vi "Periodic Tasks.vi"(8 "error in":errorcluster) -> ()   [LabVIEW 2019]
doc: "This VI runs in parallel to other tasks. It can contain as many user-defined periodic loops as you need. These can carry out PID or other sorts of timed response."
uses:
  <vilib>/Rock Robotics/WPI/Utilities/WPI_GetSetVariantRefNum.vi
  Robot Global Data.vi
  <vilib>/addons/control/pid/pid.llb/PID (DBL).vi
  <vilib>/Rock Robotics/Network Tables/NT Write Numeric Array.vi
  <vilib>/Rock Robotics/Network Tables/NT Write Number.vi
  <vilib>/Rock Robotics/Network Tables/NT Write Boolean.vi
  Secret_Control_Library_Protected/Secret_Control_Library_Protected.lvlib
  <vilib>/addons/control/pid/NI_PID_pid.lvlib
  <vilib>/Rock Robotics/WPI/ThirdParty/JAS_Junk/TrajLib/Trajectory_Library.lvlib
panel:
  in  "Speed PID":T1={"proportional gain (Kc)"=0.6, "integral time (Ti, min)"=0.015, "derivative time (Td, min)"=0.0} {"derivative time (Td, min)" format="%.3f"; "integral time (Ti, min)" format="%.3f"; "proportional gain (Kc)" format="%.3f"}
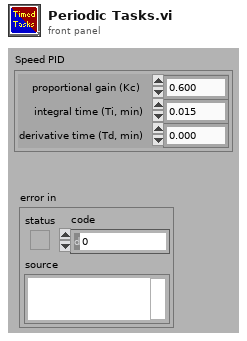
[diagram p1: front panel]
types:
  T1 = cluster{"proportional gain (Kc)":dbl, "integral time (Ti, min)":dbl, "derivative time (Td, min)":dbl}
  T2 = typedef "WPI_EncoderDevRef.ctl" = cluster{"DevStatus":errorcluster, "EncoderIndex":T3, "CounterIndex":T4, "DistancePerCount":dbl, "Decoding Type":T5}
  T3 = typedef "FPGA_EncoderIdx.ctl" = enum8{"Enc 0", "Enc 1", "Enc 2", "Enc 3", "Enc 4", "Enc 5", "Enc 6", "Enc 7", "Invalid"}
  T4 = typedef "FPGA_CounterCtrSystemIndex.ctl" = enum8{"Ctr 0", "Ctr 1", "Ctr 2", "Ctr 3", "Ctr 4", "Ctr 5", "Ctr 6", "Ctr 7", "Invalid"}
  T5 = typedef "WPI_EncoderType.ctl" = enum16{"1x", "2x", "4x"}
  T6 = typedef "WPI_GyroDevRef.ctl" = cluster{"DevStatus":errorcluster, "Analog Channel":T7, "Gain (VoltsPerDegree/Second)":dbl, "Gyro Type":enum16{"Analog", "XRS450"}, "Handle":i32, "SPI Bus":T8, "Device Found":bool, "Sample Rate":dbl, "Calibrate On Open":bool, "Offset":dbl}
  T7 = typedef "FPGA_AIChannel.ctl" = enum8{"AI 0", "AI 1", "AI 2", "AI 3", "AI MXP 0", "AI MXP 1", "AI MXP 2", "AI MXP 3", "Invalid"}
  T8 = typedef "spi_bus.ctl" = enum16{"SPI On-Board, CS0", "SPI On-Board, CS1", "SPI On-Board, CS2", "SPI On-Board, CS3", "SPI MXP", "Invalid"}
  T9 = typedef "WPI_RobotDriveDevRef.ctl" = cluster{"DevStatus":errorcluster, "Motors[]":T10[], "Square Inputs":bool, "Max Output":dbl}
  T10 = typedef "WPI_MotorControlDeviceRef.ctl" = cluster{"DeviceStatus":errorcluster, "Type":T11, "PWM":cluster{"PWM Channel":T12, "DeadBand":T13}, "CAN":cluster{"Device Number":u8, "SetOutput VI Ref":variant, "GetOutput VI Ref":variant, "Enable VI Ref":variant, "Disable VI Ref":variant, "Data":variant}, "Invert":bool, "DIO PWM":cluster{"PWM \"Enable\" Channel":T12, "DIOChannel":T14, "PWM Rate":dbl}}
  T11 = typedef "WPI_MotorControlType.ctl" = enum16{"PWM", "CAN", "DIO PWM"}
  T12 = typedef "FPGA_DIOPWMChannel.ctl" = enum8{"PWM 0", "PWM 1", "PWM 2", "PWM 3", "PWM 4", "PWM 5", "PWM 6", "PWM 7", "PWM 8", "PWM 9", "PWM MXP 0", "PWM MXP 1", "PWM MXP 2", "PWM MXP 3", "PWM MXP 4", "PWM MXP 5", "PWM MXP 6", "PWM MXP 7", "PWM MXP 8", "PWM MXP 9", "Invalid"}
  T13 = typedef "WPI_PWMDeadband.ctl" = cluster{"Name":string, "maxPositivePwm":i32, "minPositivePwm":i32, "centerPwm":i32, "maxNegativePwm":i32, "minNegativePwm":i32, "angularRange":u16}
  T14 = typedef "FPGA_DIOChannel.ctl" = enum8{"DIO 0", "DIO 1", "DIO 2", "DIO 3", "DIO 4", "DIO 5", "DIO 6", "DIO 7", "DIO 8", "DIO 9", "DIO MXP 0", "DIO MXP 1", "DIO MXP 2", "DIO MXP 3", "DIO MXP 4", "DIO MXP 5", "DIO MXP 6", "DIO MXP 7", "DIO MXP 8", "DIO MXP 9", "DIO MXP 10", "DIO MXP 11", "DIO MXP 12", "DIO MXP 13", "DIO MXP 14", "DIO MXP 15", "SPI Port CS1", "SPI Port CS2", "SPI Port CS3", "SPI Port MISO", "SPI Port MOSI", "Invalid"}
  T15 = typedef "Trajectory_Library.lvlib/SIMPLE_MOTOR_FF.ctl" = cluster{"Ks":dbl, "Kv":dbl, "Ka":dbl}
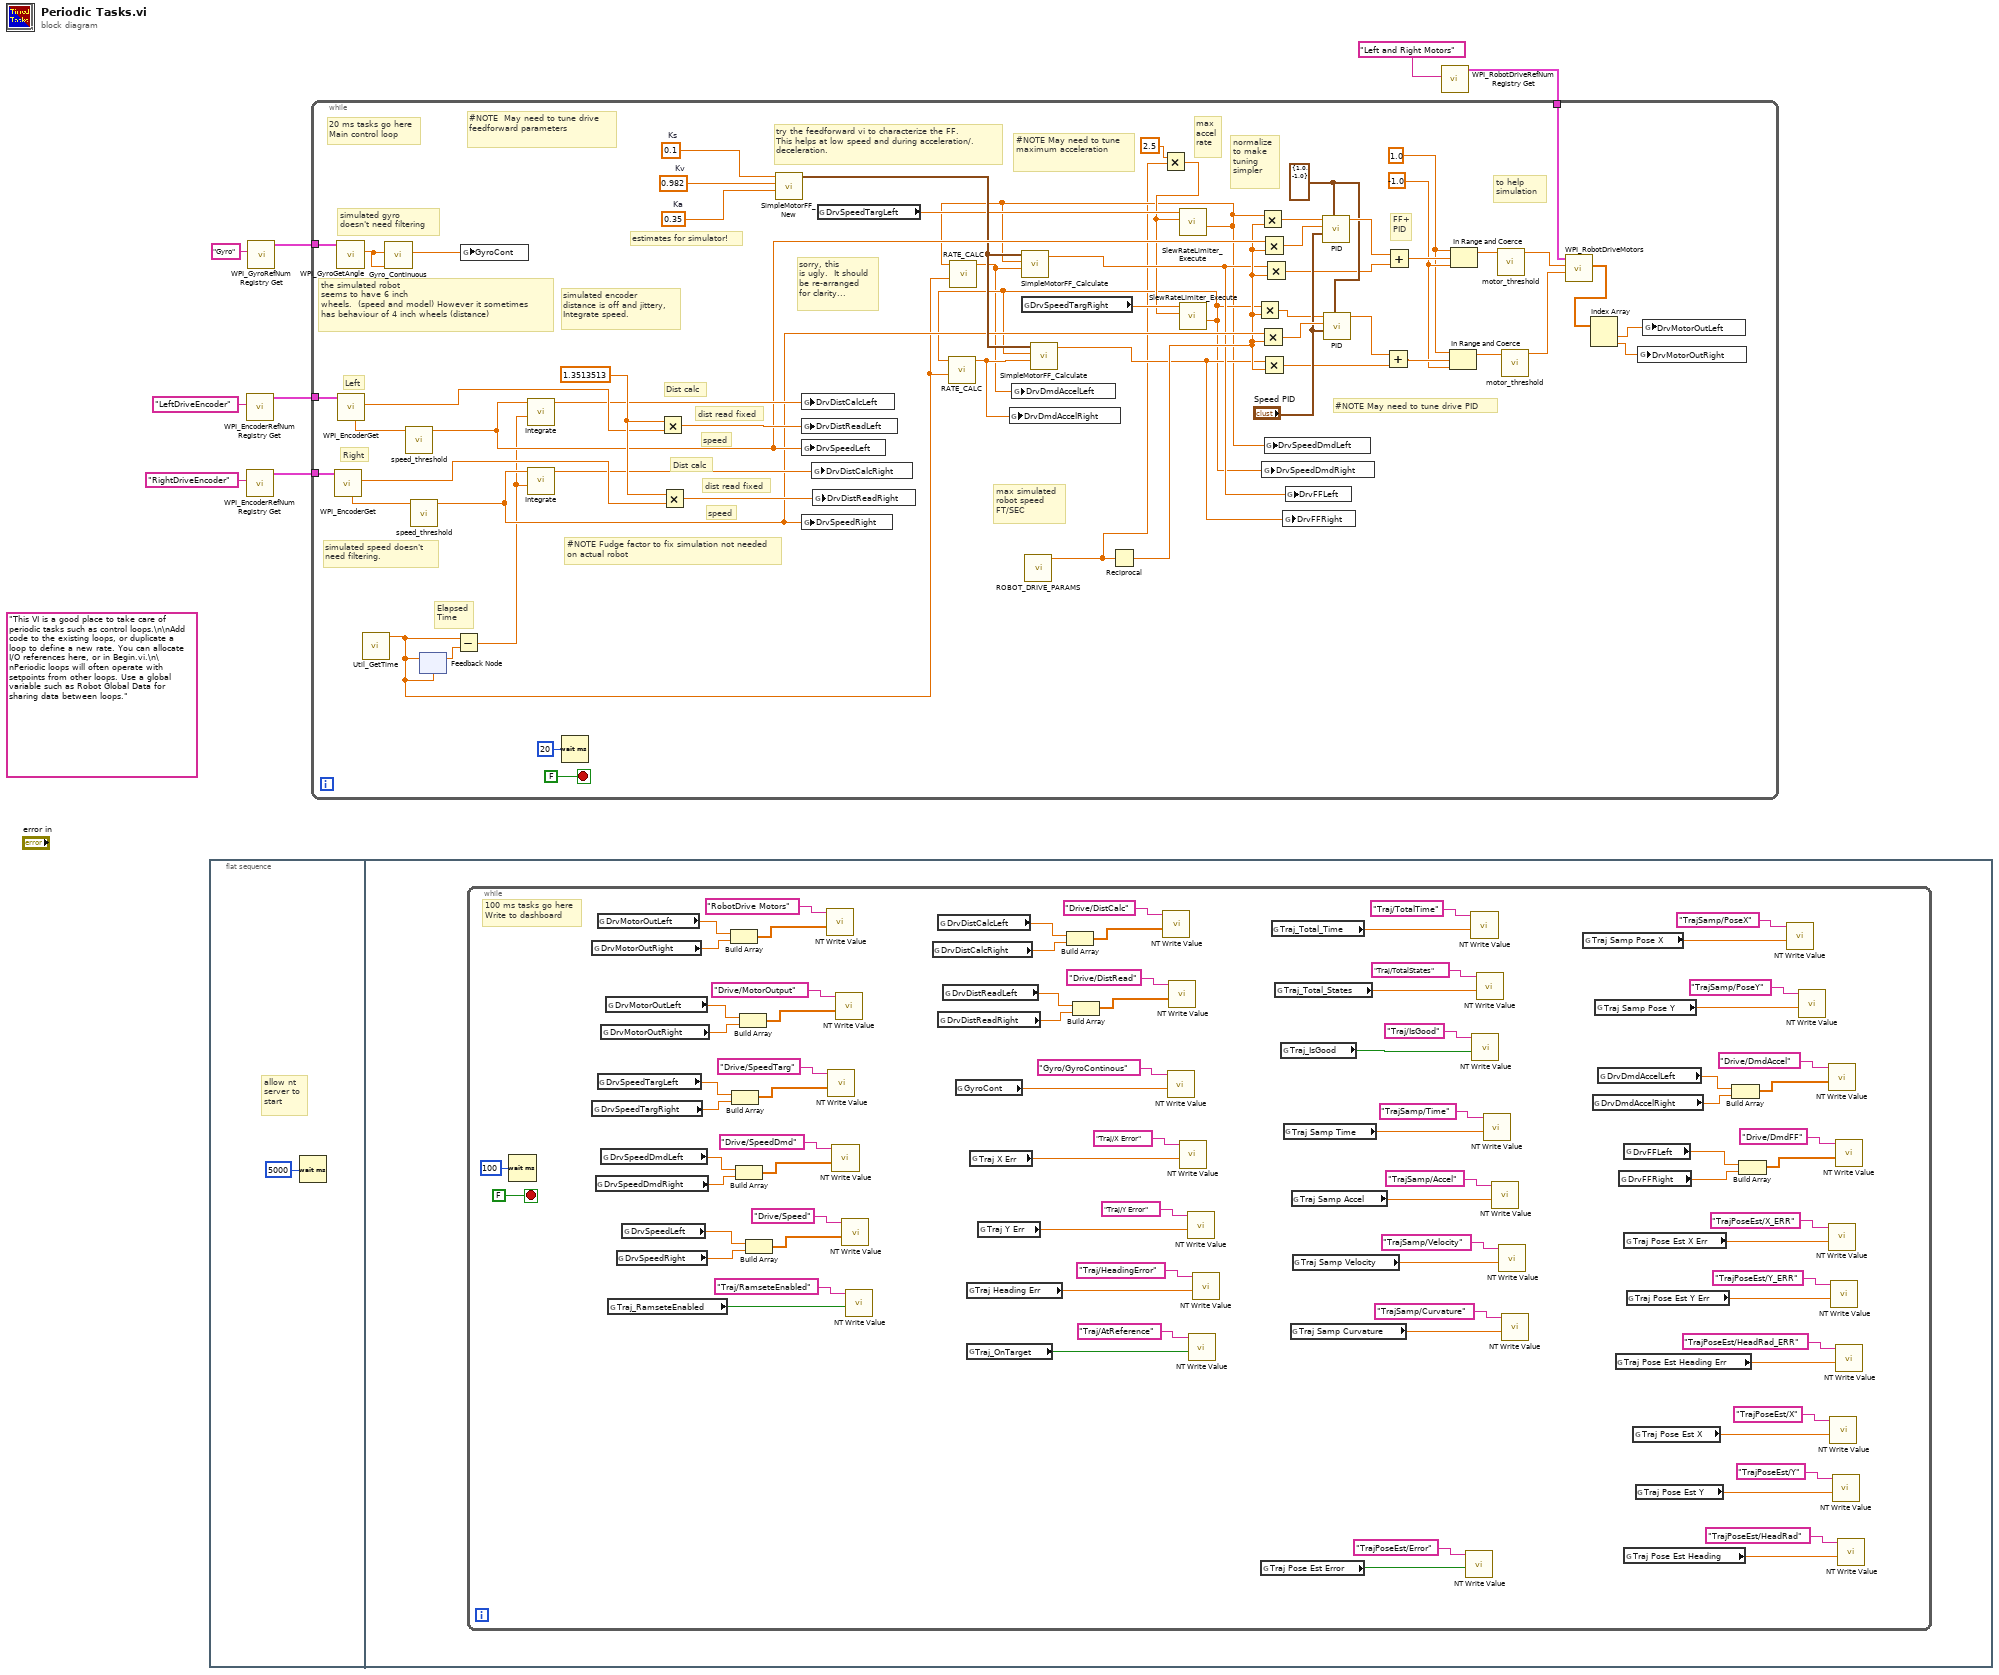
[diagram p0: block diagram]
diagram:
  (unwired) "This VI is a good place to take care of periodic tasks such as control loops.\n\nAdd code to the existing loops, or duplicate a loop to define a new rate. You can allocate I/O references here, or in Begin.vi.\n\nPeriodic loops will often operate with setpoints from other loops. Use a global variable such as Robot Global Data for sharing data between loops."
  n1 = flat-sequence {
    frame #0 {
      # "allow nt\nserver to \nstart"
      n2 = Wait (ms)(milliseconds to wait=u32 5000) -> ()  [unwired: 1 out]
    }
    frame #1 {
      n3 = while {
        stop <- FALSE stop-if-true
        # "100 ms tasks go here\nWrite to dashboard"
        n4 = Wait (ms)(milliseconds to wait=u32 100) -> ()  [unwired: 1 out]
        n5 = global read "Robot Global Data.vi" "DrvMotorOutRight"() -> (w88:dbl)
        n6 = global read "Robot Global Data.vi" "DrvSpeedTargRight"() -> (w80:dbl)
        n7 = global read "Robot Global Data.vi" "DrvSpeedDmdRight"() -> (w76:dbl)
        n8 = global read "Robot Global Data.vi" "DrvMotorOutLeft"() -> (w89:dbl)
        n9 = global read "Robot Global Data.vi" "DrvSpeedTargLeft"() -> (w81:dbl)
        n10 = global read "Robot Global Data.vi" "DrvMotorOutRight"() -> (w84:dbl)
        n11 = global read "Robot Global Data.vi" "DrvSpeedDmdLeft"() -> (w77:dbl)
        n12 = global read "Robot Global Data.vi" "DrvMotorOutLeft"() -> (w85:dbl)
        n13 = global read "Robot Global Data.vi" "Traj_RamseteEnabled"() -> (w24:bool)
        n14 = global read "Robot Global Data.vi" "DrvSpeedRight"() -> (w72:dbl)
        n15 = global read "Robot Global Data.vi" "DrvSpeedLeft"() -> (w73:dbl)
        n16 = Build Array(w89, w88) -> (w87:dbl[])
        n17 = Build Array(w81, w80) -> (w79:dbl[])
        n18 = Build Array(w77, w76) -> (w75:dbl[])
        n19 = Build Array(w85, w84) -> (w83:dbl[])
        n20 = Build Array(w73, w72) -> (w71:dbl[])
        n21 = call-poly <vilib>:"NT Write Value.vi"("Numeric Array"=w87, "Name"="RobotDrive Motors") -> ()  [unwired: 9 in, 1 out]
        n22 = call-poly <vilib>:"NT Write Value.vi"("Numeric Array"=w79, "Name"="Drive/SpeedTarg") -> ()  [unwired: 9 in, 1 out]
        n23 = call-poly <vilib>:"NT Write Value.vi"("Numeric Array"=w75, "Name"="Drive/SpeedDmd") -> ()  [unwired: 9 in, 1 out]
        n24 = call-poly <vilib>:"NT Write Value.vi"("Numeric Array"=w83, "Name"="Drive/MotorOutput") -> ()  [unwired: 9 in, 1 out]
        n25 = call-poly <vilib>:"NT Write Value.vi"("Numeric Array"=w71, "Name"="Drive/Speed") -> ()  [unwired: 9 in, 1 out]
        n26 = call-poly <vilib>:"NT Write Value.vi"("Boolean"=w24, "Name"="Traj/RamseteEnabled") -> ()  [unwired: 9 in, 1 out]
        n27 = global read "Robot Global Data.vi" "DrvDistCalcRight"() -> (w68:dbl)
        n28 = global read "Robot Global Data.vi" "DrvDistCalcLeft"() -> (w69:dbl)
        n29 = global read "Robot Global Data.vi" "DrvDistReadRight"() -> (w64:dbl)
        n30 = global read "Robot Global Data.vi" "DrvDistReadLeft"() -> (w65:dbl)
        n31 = global read "Robot Global Data.vi" "GyroCont"() -> (w60:dbl)
        n32 = global read "Robot Global Data.vi" "Traj Heading Err"() -> (w54:dbl)
        n33 = global read "Robot Global Data.vi" "Traj_OnTarget"() -> (w52:bool)
        n34 = global read "Robot Global Data.vi" "Traj X Err"() -> (w58:dbl)
        n35 = global read "Robot Global Data.vi" "Traj Y Err"() -> (w56:dbl)
        n36 = Build Array(w69, w68) -> (w67:dbl[])
        n37 = Build Array(w65, w64) -> (w63:dbl[])
        n38 = call-poly <vilib>:"NT Write Value.vi"("Numeric Array"=w67, "Name"="Drive/DistCalc") -> ()  [unwired: 9 in, 1 out]
        n39 = call-poly <vilib>:"NT Write Value.vi"("Numeric"=w60, "Name"="Gyro/GyroContinous") -> ()  [unwired: 9 in, 1 out]
        n40 = call-poly <vilib>:"NT Write Value.vi"("Numeric Array"=w63, "Name"="Drive/DistRead") -> ()  [unwired: 9 in, 1 out]
        n41 = call-poly <vilib>:"NT Write Value.vi"("Numeric"=w58, "Name"="Traj/X Error") -> ()  [unwired: 9 in, 1 out]
        n42 = call-poly <vilib>:"NT Write Value.vi"("Numeric"=w56, "Name"="Traj/Y Error") -> ()  [unwired: 9 in, 1 out]
        n43 = call-poly <vilib>:"NT Write Value.vi"("Boolean"=w52, "Name"="Traj/AtReference") -> ()  [unwired: 9 in, 1 out]
        n44 = call-poly <vilib>:"NT Write Value.vi"("Numeric"=w54, "Name"="Traj/HeadingError") -> ()  [unwired: 9 in, 1 out]
        n45 = global read "Robot Global Data.vi" "Traj Pose Est Error"() -> (w10:bool)
        n46 = global read "Robot Global Data.vi" "Traj_Total_Time"() -> (w50:dbl)
        n47 = global read "Robot Global Data.vi" "Traj_Total_States"() -> (w48:dbl)
        n48 = global read "Robot Global Data.vi" "Traj_IsGood"() -> (w46:bool)
        n49 = global read "Robot Global Data.vi" "Traj Samp Time"() -> (w44:dbl)
        n50 = global read "Robot Global Data.vi" "Traj Samp Curvature"() -> (w38:dbl)
        n51 = global read "Robot Global Data.vi" "Traj Samp Accel"() -> (w42:dbl)
        n52 = global read "Robot Global Data.vi" "Traj Samp Velocity"() -> (w40:dbl)
        n53 = call-poly <vilib>:"NT Write Value.vi"("Boolean"=w10, "Name"="TrajPoseEst/Error") -> ()  [unwired: 9 in, 1 out]
        n54 = call-poly <vilib>:"NT Write Value.vi"("Numeric"=w50, "Name"="Traj/TotalTime") -> ()  [unwired: 9 in, 1 out]
        n55 = call-poly <vilib>:"NT Write Value.vi"("Boolean"=w46, "Name"="Traj/IsGood") -> ()  [unwired: 9 in, 1 out]
        n56 = call-poly <vilib>:"NT Write Value.vi"("Numeric"=w48, "Name"="Traj/TotalStates") -> ()  [unwired: 9 in, 1 out]
        n57 = call-poly <vilib>:"NT Write Value.vi"("Numeric"=w44, "Name"="TrajSamp/Time") -> ()  [unwired: 9 in, 1 out]
        n58 = call-poly <vilib>:"NT Write Value.vi"("Numeric"=w42, "Name"="TrajSamp/Accel") -> ()  [unwired: 9 in, 1 out]
        n59 = call-poly <vilib>:"NT Write Value.vi"("Numeric"=w40, "Name"="TrajSamp/Velocity") -> ()  [unwired: 9 in, 1 out]
        n60 = call-poly <vilib>:"NT Write Value.vi"("Numeric"=w38, "Name"="TrajSamp/Curvature") -> ()  [unwired: 9 in, 1 out]
        n61 = global read "Robot Global Data.vi" "Traj Samp Pose X"() -> (w36:dbl)
        n62 = global read "Robot Global Data.vi" "DrvDmdAccelRight"() -> (w32:dbl)
        n63 = global read "Robot Global Data.vi" "Traj Samp Pose Y"() -> (w34:dbl)
        n64 = global read "Robot Global Data.vi" "DrvDmdAccelLeft"() -> (w33:dbl)
        n65 = global read "Robot Global Data.vi" "Traj Pose Est Heading Err"() -> (w18:dbl)
        n66 = global read "Robot Global Data.vi" "DrvFFRight"() -> (w28:dbl)
        n67 = global read "Robot Global Data.vi" "DrvFFLeft"() -> (w29:dbl)
        n68 = global read "Robot Global Data.vi" "Traj Pose Est X Err"() -> (w22:dbl)
        n69 = global read "Robot Global Data.vi" "Traj Pose Est Heading"() -> (w12:dbl)
        n70 = global read "Robot Global Data.vi" "Traj Pose Est Y Err"() -> (w20:dbl)
        n71 = global read "Robot Global Data.vi" "Traj Pose Est X"() -> (w16:dbl)
        n72 = global read "Robot Global Data.vi" "Traj Pose Est Y"() -> (w14:dbl)
        n73 = Build Array(w33, w32) -> (w31:dbl[])
        n74 = Build Array(w29, w28) -> (w27:dbl[])
        n75 = call-poly <vilib>:"NT Write Value.vi"("Numeric"=w36, "Name"="TrajSamp/PoseX") -> ()  [unwired: 9 in, 1 out]
        n76 = call-poly <vilib>:"NT Write Value.vi"("Numeric"=w34, "Name"="TrajSamp/PoseY") -> ()  [unwired: 9 in, 1 out]
        n77 = call-poly <vilib>:"NT Write Value.vi"("Numeric Array"=w31, "Name"="Drive/DmdAccel") -> ()  [unwired: 9 in, 1 out]
        n78 = call-poly <vilib>:"NT Write Value.vi"("Numeric"=w22, "Name"="TrajPoseEst/X_ERR") -> ()  [unwired: 9 in, 1 out]
        n79 = call-poly <vilib>:"NT Write Value.vi"("Numeric"=w16, "Name"="TrajPoseEst/X") -> ()  [unwired: 9 in, 1 out]
        n80 = call-poly <vilib>:"NT Write Value.vi"("Numeric"=w20, "Name"="TrajPoseEst/Y_ERR") -> ()  [unwired: 9 in, 1 out]
        n81 = call-poly <vilib>:"NT Write Value.vi"("Numeric"=w14, "Name"="TrajPoseEst/Y") -> ()  [unwired: 9 in, 1 out]
        n82 = call-poly <vilib>:"NT Write Value.vi"("Numeric Array"=w27, "Name"="Drive/DmdFF") -> ()  [unwired: 9 in, 1 out]
        n83 = call-poly <vilib>:"NT Write Value.vi"("Numeric"=w18, "Name"="TrajPoseEst/HeadRad_ERR") -> ()  [unwired: 9 in, 1 out]
        n84 = call-poly <vilib>:"NT Write Value.vi"("Numeric"=w12, "Name"="TrajPoseEst/HeadRad") -> ()  [unwired: 9 in, 1 out]
      }
    }
  }
  n85 = call <vilib>:"WPI_EncoderRefNum Registry Get.vi"("refnum name"="LeftDriveEncoder") -> ("EncoderDevRef"=w6:T2)  [unwired: 9 in, 1 out]
  n86 = call <vilib>:"WPI_EncoderRefNum Registry Get.vi"("refnum name"="RightDriveEncoder") -> ("EncoderDevRef"=w7:T2)  [unwired: 9 in, 1 out]
  n87 = call <vilib>:"WPI_GyroRefNum Registry Get.vi"("refnum name"="Gyro") -> ("GyroDevRef"=w2:T6)  [unwired: 9 in, 1 out]
  n88 = call <vilib>:"WPI_RobotDriveRefNum Registry Get.vi"("refnum name"="Left and Right Motors") -> ("RobotDriveDevRef"=w1:T9)  [unwired: 1 in, 9 out]
  n89 = while {
    tunnel: w7 -> [w145]
    tunnel: w6 -> [w144]
    tunnel: w2 -> [w142]
    tunnel: w1 -> [w128]
    stop <- FALSE stop-if-true
    w111 = 0.35  # Ka
    w112 = 0.982  # Kv
    w113 = 0.1  # Ks
    w137 = -1.0 ("lower limit")
    w136 = 1.0 ("upper limit")
    w134 = cluster{"output high":dbl, "output low":dbl} {"output high"=1.0, "output low"=-1.0} ("output range")
    w148 = 1.3513513
    # "#NOTE Fudge factor to fix simulation not needed on actual robot"
    # "#NOTE May need to tune maximum acceleration"
    # "#NOTE May need to tune drive PID"
    # "#NOTE  May need to tune drive feedforward parameters"
    # "Elapsed\nTime"
    # "estimates for simulator!"
    # "sorry, this\nis ugly.  It should\nbe re-arranged\nfor clarity..."
    # "try the feedforward vi to characterize the FF.\nThis helps at low speed and during acceleration/.\ndeceleration."
    # "to help\nsimulation"
    # "simulated speed doesn't\nneed filtering."
    # "max simulated\nrobot speed\nFT/SEC"
    # "max\naccel\nrate"
    # "normalize\nto make\ntuning\nsimpler"
    # "FF+\nPID"
    # "simulated gyro \ndoesn't need filtering"
    # "Right"
    # "Left"
    # "the simulated robot\nseems to have 6 inch\nwheels.  (speed and model) However it sometimes\nhas behaviour of 4 inch wheels (distance)"
    # "speed"
    # "dist read fixed"
    # "Dist calc"
    # "speed"
    # "dist read fixed"
    # "Dist calc"
    # "simulated encoder\ndistance is off and jittery,\nIntegrate speed."
    # "20 ms tasks go here\nMain control loop"
    n90 = call <vilib>:"WPI_EncoderGet.vi"("EncoderDevRef"=w145) -> ("Distance"=w146:dbl, "Rate"=w119:dbl)  [unwired: 5 in, 4 out]
    n91 = call <vilib>:"WPI_GyroGetAngle.vi"("GyroDevRef"=w142) -> ("Angle"=w143:dbl)  [unwired: 6 in, 4 out]
    n92 = call <vilib>:"WPI_EncoderGet.vi"("EncoderDevRef"=w144) -> ("Distance"=w147:dbl, "Rate"=w120:dbl)  [unwired: 5 in, 4 out]
    n93 = call <vilib>:"Util_GetTime.vi"() -> ("FPGA_Time_Seconds"=w93:dbl)  [unwired: 10 in, 1 out]
    n94 = call "Gyro_Continuous.vi"("GyroInitial"=w143, "GyroInput"=w143) -> ("GyroContinuous"=w114:dbl)  [unwired: 9 in]
    n95 = call "speed_threshold.vi"("SPEED IN"=w120) -> ("SPEED OUT"=w110:dbl)  [unwired: 10 in]
    n96 = call "speed_threshold.vi"("SPEED IN"=w119) -> ("SPEED OUT"=w108:dbl)  [unwired: 10 in]
    n97 = feedback-in #1(w93) -> ()
    n98 = feedback #1(w93) -> (w99:dbl)
    n99 = Subtract(x=w93, y=w99) -> (x-y=w98:dbl)
    n100 = global write "Robot Global Data.vi" "GyroCont"(w114) -> ()
    n101 = call "Integrate.vi"("Elapsed Sec"=w98, "Rate"=w110) -> ("DIST"=w127:dbl)  [unwired: 9 in]
    n102 = call "Integrate.vi"("Elapsed Sec"=w98, "Rate"=w108) -> ("DIST"=w125:dbl)  [unwired: 9 in]
    n103 = Wait (ms)(milliseconds to wait=u32 20) -> ()  [unwired: 1 out]
    n104 = Multiply(x=w148, y=w147) -> (x*y=w126:dbl)
    n105 = Multiply(x=w148, y=w146) -> (x*y=w124:dbl)
    n106 = call <vilib>:"SimpleMotorFF_New.vi"("Ka"=w111, "Kv"=w112, "Ks"=w113) -> ("SIMPLE_MOTOR_FF"=w109:T15)  [unwired: 8 in]
    n107 = global write "Robot Global Data.vi" "DrvDistCalcLeft"(w127) -> ()
    n108 = global write "Robot Global Data.vi" "DrvDistReadLeft"(w126) -> ()
    n109 = global write "Robot Global Data.vi" "DrvSpeedLeft"(w110) -> ()
    n110 = global write "Robot Global Data.vi" "DrvSpeedRight"(w108) -> ()
    n111 = global write "Robot Global Data.vi" "DrvDistCalcRight"(w125) -> ()
    n112 = global write "Robot Global Data.vi" "DrvDistReadRight"(w124) -> ()
    n113 = global read "Robot Global Data.vi" "DrvSpeedTargLeft"() -> (w102:dbl)
    n114 = global read "Robot Global Data.vi" "DrvSpeedTargRight"() -> (w101:dbl)
    n115 = call "ROBOT_DRIVE_PARAMS.vi"() -> ("Max Speed Ft/Sec"=w92:dbl)  [unwired: 10 in, 1 out]
    n116 = Reciprocal(x=w92) -> (1/x=w107:dbl)
    n117 = Multiply(x=2.5, y=w92) -> (x*y=w100:dbl)
    n118 = call <vilib>:"SlewRateLimiter_Execute.vi"("Rate"=w100, "Input"=w102) -> ("Output"=w94:dbl)  [unwired: 8 in, 1 out]
    n119 = call "RATE_CALC.vi"("Time"=w93, "Input"=w94) -> ("Output"=w95:dbl)  [unwired: 9 in]
    n120 = global write "Robot Global Data.vi" "DrvDmdAccelLeft"(w95) -> ()
    n121 = call <vilib>:"SimpleMotorFF_Calculate.vi"("Accel"=w95, "Vel"=w94, "SIMPLE_MOTOR_FF"=w109) -> ("FeedForward"=w104:dbl)  [unwired: 8 in]
    n122 = call <vilib>:"SlewRateLimiter_Execute.vi"("Rate"=w100, "Input"=w101) -> ("Output"=w96:dbl)  [unwired: 8 in, 1 out]
    n123 = call "RATE_CALC.vi"("Time"=w93, "Input"=w96) -> ("Output"=w97:dbl)  [unwired: 9 in]
    n124 = global write "Robot Global Data.vi" "DrvDmdAccelRight"(w97) -> ()
    n125 = call <vilib>:"SimpleMotorFF_Calculate.vi"("Accel"=w97, "Vel"=w96, "SIMPLE_MOTOR_FF"=w109) -> ("FeedForward"=w103:dbl)  [unwired: 8 in]
    n126 = Multiply(x=w96, y=w107) -> (x*y=w131:dbl)
    n127 = Multiply(x=w94, y=w107) -> (x*y=w130:dbl)
    n128 = Multiply(x=w108, y=w107) -> (x*y=w135:dbl)
    n129 = Multiply(x=w110, y=w107) -> (x*y=w132:dbl)
    n130 = Multiply(x=w103, y=w107) -> (x*y=w105:dbl)
    n131 = global write "Robot Global Data.vi" "DrvSpeedDmdRight"(w96) -> ()
    n132 = Multiply(x=w104, y=w107) -> (x*y=w106:dbl)
    n133 = global write "Robot Global Data.vi" "DrvSpeedDmdLeft"(w94) -> ()
    n134 = global write "Robot Global Data.vi" "DrvFFRight"(w103) -> ()
    n135 = global write "Robot Global Data.vi" "DrvFFLeft"(w104) -> ()
    n136 = call-poly <vilib>:"PID.vi"("output range"=w134, "PID gains"="Speed PID", "process variable"=w132, "setpoint"=w130) -> ("output"=w141:dbl)  [unwired: 6 in, 1 out]
    n137 = call-poly <vilib>:"PID.vi"("output range"=w134, "PID gains"="Speed PID", "process variable"=w135, "setpoint"=w131) -> ("output"=w139:dbl)  [unwired: 6 in, 1 out]
    n138 = Add(x=w139, y=w105) -> (x+y=w138:dbl)
    n139 = Add(x=w141, y=w106) -> (x+y=w140:dbl)
    n140 = In Range and Coerce(upper limit=w136, x=w138, lower limit=w137) -> (coerced(x)=w116:dbl)  [unwired: 1 out]
    n141 = In Range and Coerce(upper limit=w136, x=w140, lower limit=w137) -> (coerced(x)=w117:dbl)  [unwired: 1 out]
    n142 = call "motor_threshold.vi"("motor in"=w117) -> ("motor out"=w118:dbl)  [unwired: 10 in]
    n143 = call "motor_threshold.vi"("motor in"=w116) -> ("motor out"=w115:dbl)  [unwired: 10 in]
    n144 = call <vilib>:"WPI_RobotDriveMotors.vi"("RightSpeed"=w115, "LeftSpeed"=w118, "RobotDriveDevRef"=w128) -> ("Motor Values"=w123:dbl[])  [unwired: 6 in, 2 out]
    n145 = Index Array(array=w123) -> (element #1=w122:dbl, element #2=w121:dbl)  [unwired: 2 in]
    n146 = global write "Robot Global Data.vi" "DrvMotorOutRight"(w121) -> ()
    n147 = global write "Robot Global Data.vi" "DrvMotorOutLeft"(w122) -> ()
  }
